vi "nanocal -- nuclear schottky fit V8.vi"() -> ()   [LabVIEW 2021] (continued)
   ,  \"mm3\" -> 0.162147674837   ,  \"T\" -> 0.178000000000   ,  \"B\" -> 8.000000000000   ,  \"θ\" -> 90.000000000000   ,  \"Reoff\" -> 0.000000000000   ,  \"Imoff\" -> 0.000000000000   ,  \"στ1\" -> 0.000050446338   ,  \"στS\" -> 0.000029155358   ,  \"στN\" -> 0.000054402622   ,  \"τ11 \" -> 0.000000000000   ,  \"τ12\" -> 0.000000000000   ,  \"τ22\" -> 0.000000000000   ,  \"τN1\" -> 0.000000000000   ,  \"τN2\" -> 0.000000000000   ,  \"σηlogτ1 \" -> 0.161173739457   ,  \"σηlogτS\" -> 0.007924149958   ,  \"σηlogτN\" -> 0.155365649649   ,  \"σlogτ1\" -> 0.001613673870   ,  \"σlogτS\" -> 0.000552329615   ,  \"σlogτN\" -> 0.000864292135   ,  \"σητ1\" -> 0.005038580001   ,  \"σητS \" -> 0.000418285426   ,  \"σητN\" -> 0.009779446506    |>   , \n\"IDS0348_210906_RAW_cal__sam_\" ->   <|    \"ζ\" -> 0.135783247929   ,  \"τ1\" -> 0.037121050091   ,  \"τS\" -> 0.079201640502   ,  \"τN\" -> 0.079201640502   ,  \"τC\" -> 0.001474311209   ,  \"κ0\" -> 0.000000000894   ,  \"mm1\" -> 0.000173730712   ,  \"mm2\" -> 0.016810842330   ,  \"mm3\" -> 0.201522581240   ,  \"T\" -> 0.178000000000   ,  \"B\" -> 8.000000000000   ,  \"θ\" -> 90.000000000000   ,  \"Reoff\" -> -29680722.891566276600   ,  \"Imoff\" -> 0.000000000000   ,  \"στ1\" -> 0.000000000000   ,  \"στS\" -> 0.000000000000   ,  \"στN\" -> 0.000000000000   ,  \"τ11 \" -> 0.000000000000   ,  \"τ12\" -> 0.000000000000   ,  \"τ22\" -> 0.000000000000   ,  \"τN1\" -> 0.000000000000   ,  \"τN2\" -> 0.000000000000   ,  \"σηlogτ1 \" -> 0.000000000000   ,  \"σηlogτS\" -> 0.000000000000   ,  \"σηlogτN\" -> 0.000000000000   ,  \"σlogτ1\" -> 0.000000000000   ,  \"σlogτS\" -> 0.000000000000   ,  \"σlogτN\" -> 0.000000000000   ,  \"σητ1\" -> 0.000000000000   ,  \"σητS \" -> 0.000000000000   ,  \"σητN\" -> 0.000000000000    |>   , \n\"IDS0349_210906_RAW_cal__ref_\" ->   <|    \"ζ\" -> 0.197057469427   ,  \"τ1\" -> 0.029613620558   ,  \"τS\" -> 0.050911815815   ,  \"τN\" -> 0.036816442025   ,  \"τC\" -> 0.000965034060   ,  \"κ0\" -> 0.000000001032   ,  \"mm1\" -> 0.000156774968   ,  \"mm2\" -> 0.015211417778   ,  \"mm3\" -> 0.120226228200   ,  \"T\" -> 0.200000000000   ,  \"B\" -> 8.000000000000   ,  \"θ\" -> 90.000000000000   ,  \"Reoff\" -> 0.000000000000   ,  \"Imoff\" -> 0.000000000000   ,  \"στ1\" -> 0.000057169127   ,  \"στS\" -> 0.000023609008   ,  \"στN\" -> 0.000037318979   ,  \"τ11 \" -> 0.000000000000   ,  \"τ12\" -> 0.000000000000   ,  \"τ22\" -> 0.000000000000   ,  \"τN1\" -> 0.000000000000   ,  \"τN2\" -> 0.000000000000   ,  \"σηlogτ1 \" -> 0.161376688793   ,  \"σηlogτS\" -> 0.005816962816   ,  \"σηlogτN\" -> 0.148995950079   ,  \"σlogτ1\" -> 0.001930501090   ,  \"σlogτS\" -> 0.000463723546   ,  \"σlogτN\" -> 0.001013649805   ,  \"σητ1\" -> 0.004778948029   ,  \"σητS \" -> 0.000296152139   ,  \"σητN\" -> 0.005485500758    |>   , \n\"IDS0349_210906_RAW_cal__sam_\" ->   <|    \"ζ\" -> 0.113690190882   ,  \"τ1\" -> 0.032691214581   ,  \"τS\" -> 0.068786957350   ,  \"τN\" -> 0.048058332081   ,  \"τC\" -> 0.001613875480   ,  \"κ0\" -> 0.000000001156   ,  \"mm1\" -> 0.000161675745   ,  \"mm2\" -> 0.017372504664   ,  \"mm3\" -> 0.146900362342   ,  \"T\" -> 0.200000000000   ,  \"B\" -> 8.000000000000   ,  \"θ\" -> 90.000000000000   ,  \"Reoff\" -> -14590361.445783138300   ,  \"Imoff\" -> 0.000000000000   ,  \"στ1\" -> 0.000000000000   ,  \"στS\" -> 0.000000000000   ,  \"στN\" -> 0.000000000000   ,  \"τ11 \" -> 0.000000000000   ,  \"τ12\" -> 0.000000000000   ,  \"τ22\" -> 0.000000000000   ,  \"τN1\" -> 0.000000000000   ,  \"τN2\" -> 0.000000000000   ,  \"σηlogτ1 \" -> 0.000000000000   ,  \"σηlogτS\" -> 0.000000000000   ,  \"σηlogτN\" -> 0.000000000000   ,  \"σlogτ1\" -> 0.000000000000   ,  \"σlogτS\" -> 0.000000000000   ,  \"σlogτN\" -> 0.000000000000   ,  \"σητ1\" -> 0.000000000000   ,  \"σητS \" -> 0.000000000000   ,  \"σητN\" -> 0.000000000000    |>   , \n\"IDS0350_210906_RAW_cal__ref_\" ->   <|    \"ζ\" -> 0.116383968065   ,  \"τ1\" -> 0.022837025685   ,  \"τS\" -> 0.041355624864   ,  \"τN\" -> 0.016243225582   ,  \"τC\" -> 0.001144746242   ,  \"κ0\" -> 0.000000001355   ,  \"mm1\" -> 0.000116736213   ,  \"mm2\" -> 0.014664448269   ,  \"mm3\" -> 0.073503020661   ,  \"T\" -> 0.260000000000   ,  \"B\" -> 8.000000000000   ,  \"θ\" -> 90.000000000000   ,  \"Reoff\" -> 0.000000000000   ,  \"Imoff\" -> 0.000000000000   ,  \"στ1\" -> 0.000027906584   ,  \"στS\" -> 0.000007380086   ,  \"στN\" -> 0.000010191855   ,  \"τ11 \" -> 0.000000000000   ,  \"τ12\" -> 0.000000000000   ,  \"τ22\" -> 0.000000000000   ,  \"τN1\" -> 0.000000000000   ,  \"τN2\" -> 0.000000000000   ,  \"σηlogτ1 \" -> 0.162256483080   ,  \"σηlogτS\" -> 0.003668520899   ,  \"σηlogτN\" -> 0.144232966841   ,  \"σlogτ1\" -> 0.001221988557   ,  \"σlogτS\" -> 0.000178454219   ,  \"σlogτN\" -> 0.000627452654   ,  \"σητ1\" -> 0.003705455472   ,  \"σητS \" -> 0.000151713974   ,  \"σητN\" -> 0.002342808617    |>   , \n\"IDS0350_210906_RAW_cal__sam_\" ->   <|    \"ζ\" -> 0.071614468485   ,  \"τ1\" -> 0.024327525692   ,  \"τS\" -> 0.055056024171   ,  \"τN\" -> 0.019709093999   ,  \"τC\" -> 0.001754398678   ,  \"κ0\" -> 0.000000001497   ,  \"mm1\" -> 0.000114067222   ,  \"mm2\" -> 0.016460052715   ,  \"mm3\" -> 0.089627186802   ,  \"T\" -> 0.260000000000   ,  \"B\" -> 8.000000000000   ,  \"θ\" -> 90.000000000000   ,  \"Reoff\" -> -10063253.012048184900   ,  \"Imoff\" -> 0.000000000000   ,  \"στ1\" -> 0.000000000000   ,  \"στS\" -> 0.000000000000   ,  \"στN\" -> 0.000000000000   ,  \"τ11 \" -> 0.000000000000   ,  \"τ12\" -> 0.000000000000   ,  \"τ22\" -> 0.000000000000   ,  \"τN1\" -> 0.000000000000   ,  \"τN2\" -> 0.000000000000   ,  \"σηlogτ1 \" -> 0.000000000000   ,  \"σηlogτS\" -> 0.000000000000   ,  \"σηlogτN\" -> 0.000000000000   ,  \"σlogτ1\" -> 0.000000000000   ,  \"σlogτS\" -> 0.000000000000   ,  \"σlogτN\" -> 0.000000000000   ,  \"σητ1\" -> 0.000000000000   ,  \"σητS \" -> 0.000000000000   ,  \"σητN\" -> 0.000000000000    |>   , \n\"IDS0351_210906_RAW_cal__ref_\" ->   <|    \"ζ\" -> 0.080064937947   ,  \"τ1\" -> 0.017296327437   ,  \"τS\" -> 0.036479707086   ,  \"τN\" -> 0.008116806938   ,  \"τC\" -> 0.001346314476   ,  \"κ0\" -> 0.000000001766   ,  \"mm1\" -> 0.000096730306   ,  \"mm2\" -> 0.013119572666   ,  \"mm3\" -> 0.053593470093   ,  \"T\" -> 0.310000000000   ,  \"B\" -> 8.000000000000   ,  \"θ\" -> 90.000000000000   ,  \"Reoff\" -> 0.000000000000   ,  \"Imoff\" -> 0.000000000000   ,  \"στ1\" -> 0.000031102743   ,  \"στS\" -> 0.000006077841   ,  \"στN\" -> 0.000007305969   ,  \"τ11 \" -> 0.000000000000   ,  \"τ12\" -> 0.000000000000   ,  \"τ22\" -> 0.000000000000   ,  \"τN1\" -> 0.000000000000   ,  \"τN2\" -> 0.000000000000   ,  \"σηlogτ1 \" -> 0.176104217691   ,  \"σηlogτS\" -> 0.002693810692   ,  \"σηlogτN\" -> 0.144358868609   ,  \"σlogτ1\" -> 0.001798228177   ,  \"σlogτS\" -> 0.000166608817   ,  \"σlogτN\" -> 0.000900103833   ,  \"σητ1\" -> 0.003045956212   ,  \"σητS \" -> 0.000098269425   ,  \"σητN\" -> 0.001171733066    |>   , \n\"IDS0351_210906_RAW_cal__sam_\" ->   <|    \"ζ\" -> 0.049866383839   ,  \"τ1\" -> 0.023285662985   ,  \"τS\" -> 0.049370833464   ,  \"τN\" -> 0.009866658615   ,  \"τC\" -> 0.002153040267   ,  \"κ0\" -> 0.000000001928   ,  \"mm1\" -> 0.000098362318   ,  \"mm2\" -> 0.018063601956   ,  \"mm3\" -> 0.069468190575   ,  \"T\" -> 0.310000000000   ,  \"B\" -> 8.000000000000   ,  \"θ\" -> 90.000000000000   ,  \"Reoff\" -> -5536144.578313261270   ,  \"Imoff\" -> 0.000000000000   ,  \"στ1\" -> 0.000000000000   ,  \"στS\" -> 0.000000000000   ,  \"στN\" -> 0.000000000000   ,  \"τ11 \" -> 0.000000000000   ,  \"τ12\" -> 0.000000000000   ,  \"τ22\" -> 0.000000000000   ,  \"τN1\" -> 0.000000000000   ,  \"τN2\" -> 0.000000000000   ,  \"σηlogτ1 \" -> 0.000000000000   ,  \"σηlogτS\" -> 0.000000000000   ,  \"σηlogτN\" -> 0.000000000000   ,  \"σlogτ1\" -> 0.000000000000   ,  \"σlogτS\" -> 0.000000000000   ,  \"σlogτN\" -> 0.000000000000   ,  \"σητ1\" -> 0.000000000000   ,  \"σητS \" -> 0.000000000000   ,  \"σητN\" -> 0.000000000000    |>   , \n\"IDS0352_210906_RAW_cal__ref_\" ->   <|    \"ζ\" -> 0.060178216595   ,  \"τ1\" -> 0.015538327560   ,  \"τS\" -> 0.033922393417   ,  \"τN\" -> 0.005018769313   ,  \"τC\" -> 0.001649636137   ,  \"κ0\" -> 0.000000002110   ,  \"mm1\" -> 0.000089741441   ,  \"mm2\" -> 0.012788298806   ,  \"mm3\" -> 0.045594495906   ,  \"T\" -> 0.360000000000   ,  \"B\" -> 8.000000000000   ,  \"θ\" -> 90.000000000000   ,  \"Reoff\" -> 0.000000000000   ,  \"Imoff\" -> 0.000000000000   ,  \"στ1\" -> 0.000024762200   ,  \"στS\" -> 0.000003463726   ,  \"στN\" -> 0.000003978144   ,  \"τ11 \" -> 0.000000000000   ,  \"τ12\" -> 0.000000000000   ,  \"τ22\" -> 0.000000000000   ,  \"τN1\" -> 0.000000000000   ,  \"τN2\" -> 0.000000000000   ,  \"σηlogτ1 \" -> 0.179978131634   ,  \"σηlogτS\" -> 0.001942969644   ,  \"σηlogτN\" -> 0.143630935441   ,  \"σlogτ1\" -> 0.001593620678   ,  \"σlogτS\" -> 0.000102107372   ,  \"σlogτN\" -> 0.000792653332   ,  \"σητ1\" -> 0.002796559163   ,  \"σητS \" -> 0.000065910181   ,  \"σητN\" -> 0.000720850531    |>   , \n\"IDS0352_210906_RAW_cal__sam_\" ->   <|    \"ζ\" -> 0.036116393265   ,  \"τ1\" -> 0.020310974732   ,  \"τS\" -> 0.044594628397   ,  \"τN\" -> 0.005932938101   ,  \"τC\" -> 0.002747123875   ,  \"κ0\" -> 0.000000002292   ,  \"mm1\" -> 0.000090548575   ,  \"mm2\" -> 0.017024776182   ,  \"mm3\" -> 0.058295213810   ,  \"T\" -> 0.360000000000   ,  \"B\" -> 8.000000000000   ,  \"θ\" -> 90.000000000000   ,  \"Reoff\" -> -2518072.289156645540   ,  \"Imoff\" -> 0.000000000000   ,  \"στ1\" -> 0.000000000000   ,  \"στS\" -> 0.000000000000   ,  \"στN\" -> 0.000000000000   ,  \"τ11 \" -> 0.000000000000   ,  \"τ12\" -> 0.000000000000   ,  \"τ22\" -> 0.000000000000   ,  \"τN1\" -> 0.000000000000   ,  \"τN2\" -> 0.000000000000   ,  \"σηlogτ1 \" -> 0.000000000000   ,  \"σηlogτS\" -> 0.000000000000   ,  \"σηlogτN\" -> 0.000000000000   ,  \"σlogτ1\" -> 0.000000000000   ,  \"σlogτS\" -> 0.000000000000   ,  \"σlogτN\" -> 0.000000000000   ,  \"σητ1\" -> 0.000000000000   ,  \"σητS \" -> 0.000000000000   ,  \"σητN\" -> 0.000000000000    |>   , \n\"IDS0353_210906_RAW_cal__ref_\" ->   <|    \"ζ\" -> 0.043805011586   ,  \"τ1\" -> 0.015641832651   ,  \"τS\" -> 0.031297289619   ,  \"τN\" -> 0.002720036846   ,  \"τC\" -> 0.001830581120   ,  \"κ0\" -> 0.000000002632   ,  \"mm1\" -> 0.000072899501   ,  \"mm2\" -> 0.013753455926   ,  \"mm3\" -> 0.039153514190   ,  \"T\" -> 0.438000000000   ,  \"B\" -> 8.000000000000   ,  \"θ\" -> 90.000000000000   ,  \"Reoff\" -> 0.000000000000   ,  \"Imoff\" -> 0.000000000000   ,  \"στ1\" -> 0.000029789904   ,  \"στS\" -> 0.000002213568   ,  \"στN\" -> 0.000002569992   ,  \"τ11 \" -> 0.000000000000   ,  \"τ12\" -> 0.000000000000   ,  \"τ22\" -> 0.000000000000   ,  \"τN1\" -> 0.000000000000   ,  \"τN2\" -> 0.000000000000   ,  \"σηlogτ1 \" -> 0.171230545078   ,  \"σηlogτS\" -> 0.001043214583   ,  \"σηlogτN\" -> 0.141039696626   ,  \"σlogτ1\" -> 0.001904502144   ,  \"σlogτS\" -> 0.000070727156   ,  \"σlogτN\" -> 0.000944837375   ,  \"σητ1\" -> 0.002678359531   ,  \"σητS \" -> 0.000032649789   ,  \"σητN\" -> 0.000383633172    |>   , \n\"IDS0353_210906_RAW_cal__sam_\" ->   <|    \"ζ\" -> 0.028235631162   ,  \"τ1\" -> 0.018033623612   ,  \"τS\" -> 0.040112967891   ,  \"τN\" -> 0.003332308168   ,  \"τC\" -> 0.002994357278   ,  \"κ0\" -> 0.000000002859   ,  \"mm1\" -> 0.000076791949   ,  \"mm2\" -> 0.016073609718   ,  \"mm3\" -> 0.049549560072   ,  \"T\" -> 0.438000000000   ,  \"B\" -> 8.000000000000   ,  \"θ\" -> 90.000000000000   ,  \"Reoff\" -> -2200000.000000000000   ,  \"Imoff\" -> 0.000000000000   ,  \"στ1\" -> 0.000000000000   ,  \"στS\" -> 0.000000000000   ,  \"στN\" -> 0.000000000000   ,  \"τ11 \" -> 0.000000000000   ,  \"τ12\" -> 0.000000000000   ,  \"τ22\" -> 0.000000000000   ,  \"τN1\" -> 0.000000000000   ,  \"τN2\" -> 0.000000000000   ,  \"σηlogτ1 \" -> 0.000000000000   ,  \"σηlogτS\" -> 0.000000000000   ,  \"σηlogτN\" -> 0.000000000000   ,  \"σlogτ1\" -> 0.000000000000   ,  \"σlogτS\" -> 0.000000000000   ,  \"σlogτN\" -> 0.000000000000   ,  \"σητ1\" -> 0.000000000000   ,  \"σητS \" -> 0.000000000000   ,  \"σητN\" -> 0.000000000000    |>   , \n\"IDS0354_210906_RAW_cal__ref_\" ->   <|    \"ζ\" -> 0.034407438278   ,  \"τ1\" -> 0.012759993552   ,  \"τS\" -> 0.028549472180   ,  \"τN\" -> 0.001373973335   ,  \"τC\" -> 0.002126234468   ,  \"κ0\" -> 0.000000003285   ,  \"mm1\" -> 0.000066111743   ,  \"mm2\" -> 0.011901304001   ,  \"mm3\" -> 0.033871846896   ,  \"T\" -> 0.530000000000   ,  \"B\" -> 8.000000000000   ,  \"θ\" -> 90.000000000000   ,  \"Reoff\" -> 0.000000000000   ,  \"Imoff\" -> 0.000000000000   ,  \"στ1\" -> 0.000105401331   ,  \"στS\" -> 0.000005152140   ,  \"στN\" -> 0.000005607099   ,  \"τ11 \" -> 0.000000000000   ,  \"τ12\" -> 0.000000000000   ,  \"τ22\" -> 0.000000000000   ,  \"τN1\" -> 0.000000000000   ,  \"τN2\" -> 0.000000000000   ,  \"σηlogτ1 \" -> 0.184333164792   ,  \"σηlogτS\" -> 0.000694064017   ,  \"σηlogτN\" -> 0.142381877257   ,  \"σlogτ1\" -> 0.008260296568   ,  \"σlogτS\" -> 0.000180463565   ,  \"σlogτN\" -> 0.004080937594   ,  \"σητ1\" -> 0.002352089994   ,  \"σητS \" -> 0.000019815161   ,  \"σητN\" -> 0.000195628903    |>   , \n\"IDS0354_210906_RAW_cal__sam_\" ->   <|    \"ζ\" -> 0.022962333090   ,  \"τ1\" -> 0.020865157142   ,  \"τS\" -> 0.035948400917   ,  \"τN\" -> 0.001990138096   ,  \"τC\" -> 0.003574397791   ,  \"κ0\" -> 0.000000003542   ,  \"mm1\" -> 0.000073258085   ,  \"mm2\" -> 0.019040364220   ,  \"mm3\" -> 0.044135629011   ,  \"T\" -> 0.530000000000   ,  \"B\" -> 8.000000000000   ,  \"θ\" -> 90.000000000000   ,  \"Reoff\" -> -1700000.000000000000   ,  \"Imoff\" -> 0.000000000000   ,  \"στ1\" -> 0.000000000000   ,  \"στS\" -> 0.000000000000   ,  \"στN\" -> 0.000000000000   ,  \"τ11 \" -> 0.000000000000   ,  \"τ12\" -> 0.000000000000   ,  \"τ22\" -> 0.000000000000   ,  \"τN1\" -> 0.000000000000   ,  \"τN2\" -> 0.000000000000   ,  \"σηlogτ1 \" -> 0.000000000000   ,  \"σηlogτS\" -> 0.000000000000   ,  \"σηlogτN\" -> 0.000000000000   ,  \"σlogτ1\" -> 0.000000000000   ,  \"σlogτS\" -> 0.000000000000   ,  \"σlogτN\" -> 0.000000000000   ,  \"σητ1\" -> 0.000000000000   ,  \"σητS \" -> 0.000000000000   ,  \"σητN\" -> 0.000000000000    |>   , \n\"IDS0355_210906_RAW_cal__ref_\" ->   <|    \"ζ\" -> 0.020775547522   ,  \"τ1\" -> 0.014245155504   ,  \"τS\" -> 0.021871141548   ,  \"τN\" -> 0.000446024292   ,  \"τC\" -> 0.003241636501   ,  \"κ0\" -> 0.000000005421   ,  \"mm1\" -> 0.000057740843   ,  \"mm2\" -> 0.013715964924   ,  \"mm3\" -> 0.026493903417   ,  \"T\" -> 0.830000000000   ,  \"B\" -> 8.000000000000   ,  \"θ\" -> 90.000000000000   ,  \"Reoff\" -> 0.000000000000   ,  \"Imoff\" -> 0.000000000000   ,  \"στ1\" -> 0.000172291727   ,  \"στS\" -> 0.000002161761   ,  \"στN\" -> 0.000002696691   ,  \"τ11 \" -> 0.000000000000   ,  \"τ12\" -> 0.000000000000   ,  \"τ22\" -> 0.000000000000   ,  \"τN1\" -> 0.000000000000   ,  \"τN2\" -> 0.000000000000   ,  \"σηlogτ1 \" -> 0.152304599872   ,  \"σηlogτS\" -> 0.000189712528   ,  \"σηlogτN\" -> 0.136839329472   ,  \"σlogτ1\" -> 0.012094759326   ,  \"σlogτS\" -> 0.000098840802   ,  \"σlogτN\" -> 0.006046063343   ,  \"σητ1\" -> 0.002169602709   ,  \"σητS \" -> 0.000004149230   ,  \"σητN\" -> 0.000061033665    |>   , \n\"IDS0355_210906_RAW_cal__sam_\" ->   <|    \"ζ\" -> 0.015987398390   ,  \"τ1\" -> 0.023974349678   ,  \"τS\" -> 0.025824294014   ,  \"τN\" -> 0.000573136357   ,  \"τC\" -> 0.005688548480   ,  \"κ0\" -> 0.000000005865   ,  \"mm1\" -> 0.000073733721   ,  \"mm2\" -> 0.022561297233   ,  \"mm3\" -> 0.033847323811   ,  \"T\" -> 0.830000000000   ,  \"B\" -> 8.000000000000   ,  \"θ\" -> 90.000000000000   ,  \"Reoff\" -> -599999.999999999999   ,  \"Imoff\" -> 0.000000000000   ,  \"στ1\" -> 0.000000000000   ,  \"στS\" -> 0.000000000000   ,  \"στN\" -> 0.000000000000   ,  \"τ11 \" -> 0.000000000000   ,  \"τ12\" -> 0.000000000000   ,  \"τ22\" -> 0.000000000000   ,  \"τN1\" -> 0.000000000000   ,  \"τN2\" -> 0.000000000000   ,  \"σηlogτ1 \" -> 0.000000000000   ,  \"σηlogτS\" -> 0.000000000000   ,  \"σηlogτN\" -> 0.000000000000   ,  \"σlogτ1\" -> 0.000000000000   ,  \"σlogτS\" -> 0.000000000000   ,  \"σlogτN\" -> 0.000000000000   ,  \"σητ1\" -> 0.000000000000   ,  \"σητS \" -> 0.000000000000   ,  \"σητN\" -> 0.000000000000    |>   , \n\"IDS0359_210907_RAW_cal__ref_\" ->   <|    \"ζ\" -> 0.424845059741   ,  \"τ1\" -> 0.089321051678   ,  \"τS\" -> 0.116595960023   ,  \"τN\" -> 0.612122896867   ,  \"τC\" -> 0.001120095408   ,  \"κ0\" -> 0.000000000383   ,  \"mm1\" -> 0.000332370585   ,  \"mm2\" -> 0.013372321421   ,  \"mm3\" -> 1.115047918259   ,  \"T\" -> 0.120000000000   ,  \"B\" -> 12.000000000000   ,  \"θ\" -> 60.000000000000   ,  \"Reoff\" -> 0.000000000000   ,  \"Imoff\" -> 0.000000000000   ,  \"στ1\" -> 0.000839647107   ,  \"στS\" -> 0.000700328201   ,  \"στN\" -> 0.003352050812   ,  \"τ11 \" -> 0.000000000000   ,  \"τ12\" -> 0.000000000000   ,  \"τ22\" -> 0.000000000000   ,  \"τN1\" -> 0.000000000000   ,  \"τN2\" -> 0.000000000000   ,  \"σηlogτ1 \" -> 0.058996717292   ,  \"σηlogτS\" -> 0.003693056048   ,  \"σηlogτN\" -> 0.066658525220   ,  \"σlogτ1\" -> 0.009400327147   ,  \"σlogτS\" -> 0.006006453401   ,  \"σlogτN\" -> 0.005476107542   ,  \"σητ1\" -> 0.005269648834   ,  \"σητS \" -> 0.000430595415   ,  \"σητN\" -> 0.040803209559    |>   , \n\"IDS0359_210907_RAW_cal__sam_\" ->   <|    \"ζ\" -> 0.241762987309   ,  \"τ1\" -> 0.090301757431   ,  \"τS\" -> 0.104468976957   ,  \"τN\" -> 0.810352557873   ,  \"τC\" -> 0.001702208121   ,  \"κ0\" -> 0.000000000500   ,  \"mm1\" -> 0.000327834342   ,  \"mm2\" -> 0.009723084216   ,  \"mm3\" -> 1.217944568939   ,  \"T\" -> 0.120000000000   ,  \"B\" -> 12.000000000000   ,  \"θ\" -> 60.000000000000   ,  \"Reoff\" -> -52289156.626506023100   ,  \"Imoff\" -> 0.000000000000   ,  \"στ1\" -> 0.000000000000   ,  \"στS\" -> 0.000000000000   ,  \"στN\" -> 0.000000000000   ,  \"τ11 \" -> 0.000000000000   ,  \"τ12\" -> 0.000000000000   ,  \"τ22\" -> 0.000000000000   ,  \"τN1\" -> 0.000000000000   ,  \"τN2\" -> 0.000000000000   ,  \"σηlogτ1 \" -> 0.000000000000   ,  \"σηlogτS\" -> 0.000000000000   ,  \"σηlogτN\" -> 0.000000000000   ,  \"σlogτ1\" -> 0.000000000000   ,  \"σlogτS\" -> 0.000000000000   ,  \"σlogτN\" -> 0.000000000000   ,  \"σητ1\" -> 0.000000000000   ,  \"σητS \" -> 0.000000000000   ,  \"σητN\" -> 0.000000000000    |>   , \n\"IDS0360_210907_RAW_cal__ref_\" ->   <|    \"ζ\" -> 0.342434399581   ,  \"τ1\" -> 0.078890152129   ,  \"τS\" -> 0.062757285209   ,  \"τN\" -> 0.289377193045   ,  \"τC\" -> 0.000956599249   ,  \"κ0\" -> 0.000000000628   ,  \"mm1\" -> 0.000241931953   ,  \"mm2\" -> 0.012416031233   ,  \"mm3\" -> 0.539906225078   ,  \"T\" -> 0.150000000000   ,  \"B\" -> 12.000000000000   ,  \"θ\" -> 60.000000000000   ,  \"Reoff\" -> 0.000000000000   ,  \"Imoff\" -> 0.000000000000   ,  \"στ1\" -> 0.000259479640   ,  \"στS\" -> 0.000106061605   ,  \"στN\" -> 0.000644908503   ,  \"τ11 \" -> 0.000000000000   ,  \"τ12\" -> 0.000000000000   ,  \"τ22\" -> 0.000000000000   ,  \"τN1\" -> 0.000000000000   ,  \"τN2\" -> 0.000000000000   ,  \"σηlogτ1 \" -> 0.046682907310   ,  \"σηlogτS\" -> 0.002342389923   ,  \"σηlogτN\" -> 0.056973626918   ,  \"σlogτ1\" -> 0.003289125866   ,  \"σlogτS\" -> 0.001690028567   ,  \"σlogτN\" -> 0.002228608605   ,  \"σητ1\" -> 0.003682821660   ,  \"σητS \" -> 0.000147002032   ,  \"σητN\" -> 0.016486868235    |>   , \n\"IDS0360_210907_RAW_cal__sam_\" ->   <|    \"ζ\" -> 0.201278537585   ,  \"τ1\" -> 0.081544073952   ,  \"τS\" -> 0.088995303529   ,  \"τN\" -> 0.405130496924   ,  \"τC\" -> 0.001460686320   ,  \"κ0\" -> 0.000000000739   ,  \"mm1\" -> 0.000241947199   ,  \"mm2\" -> 0.013299947862   ,  \"mm3\" -> 0.663045584163   ,  \"T\" -> 0.150000000000   ,  \"B\" -> 12.000000000000   ,  \"θ\" -> 60.000000000000   ,  \"Reoff\" -> -39048192.771084338400   ,  \"Imoff\" -> 0.000000000000   ,  \"στ1\" -> 0.000000000000   ,  \"στS\" -> 0.000000000000   ,  \"στN\" -> 0.000000000000   ,  \"τ11 \" -> 0.000000000000   ,  \"τ12\" -> 0.000000000000   ,  \"τ22\" -> 0.000000000000   ,  \"τN1\" -> 0.000000000000   ,  \"τN2\" -> 0.000000000000   ,  \"σηlogτ1 \" -> 0.000000000000   ,  \"σηlogτS\" -> 0.000000000000   ,  \"σηlogτN\" -> 0.000000000000   ,  \"σlogτ1\" -> 0.000000000000   ,  \"σlogτS\" -> 0.000000000000   ,  \"σlogτN\" -> 0.000000000000   ,  \"σητ1\" -> 0.000000000000   ,  \"σητS \" -> 0.000000000000   ,  \"σητN\" -> 0.000000000000    |>   , \n\"IDS0361_210908_RAW_cal__ref_\" ->   <|    \"ζ\" -> 0.274843315726   ,  \"τ1\" -> 0.065669556126   ,  \"τS\" -> 0.043737045326   ,  \"τN\" -> 0.171424826572   ,  \"τC\" -> 0.000899266573   ,  \"κ0\" -> 0.000000000755   ,  \"mm1\" -> 0.000191414578   ,  \"mm2\" -> 0.011258128300   ,  \"mm3\" -> 0.329416954010   ,  \"T\" -> 0.168000000000   ,  \"B\" -> 12.000000000000   ,  \"θ\" -> 60.000000000000   ,  \"Reoff\" -> 0.000000000000   ,  \"Imoff\" -> 0.000000000000   ,  \"στ1\" -> 0.000077610156   ,  \"στS\" -> 0.000022738638   ,  \"στN\" -> 0.000144137782   ,  \"τ11 \" -> 0.000000000000   ,  \"τ12\" -> 0.000000000000   ,  \"τ22\" -> 0.000000000000   ,  \"τN1\" -> 0.000000000000   ,  \"τN2\" -> 0.000000000000   ,  \"σηlogτ1 \" -> 0.041134517971   ,  \"σηlogτS\" -> 0.001768570492   ,  \"σηlogτN\" -> 0.052373530031   ,  \"σlogτ1\" -> 0.001181828544   ,  \"σlogτS\" -> 0.000519894231   ,  \"σlogτN\" -> 0.000840822097   ,  \"σητ1\" -> 0.002701285537   ,  \"σητS \" -> 0.000077352048   ,  \"σητN\" -> 0.008978123302    |>   , \n\"IDS0361_210908_RAW_cal__sam_\" ->   <|    \"ζ\" -> 0.166104690940   ,  \"τ1\" -> 0.071049175548   ,  \"τS\" -> 0.068661809155   ,  \"τN\" -> 0.222482953546   ,  \"τC\" -> 0.001364223445   ,  \"κ0\" -> 0.000000000861   ,  \"mm1\" -> 0.000191495940   ,  \"mm2\" -> 0.014533832786   ,  \"mm3\" -> 0.397193343795   ,  \"T\" -> 0.168000000000   ,  \"B\" -> 12.000000000000   ,  \"θ\" -> 60.000000000000   ,  \"Reoff\" -> -34789156.626506023100   ,  \"Imoff\" -> 0.000000000000   ,  \"στ1\" -> 0.000000000000   ,  \"στS\" -> 0.000000000000   ,  \"στN\" -> 0.000000000000   ,  \"τ11 \" -> 0.000000000000   ,  \"τ12\" -> 0.000000000000   ,  \"τ22\" -> 0.000000000000   ,  \"τN1\" -> 0.000000000000   ,  \"τN2\" -> 0.000000000000   ,  \"σηlogτ1 \" -> 0.000000000000   ,  \"σηlogτS\" -> 0.000000000000   ,  \"σηlogτN\" -> 0.000000000000   ,  \"σlogτ1\" -> 0.000000000000   ,  \"σlogτS\" -> 0.000000000000   ,  \"σlogτN\" -> 0.000000000000   ,  \"σητ1\" -> 0.000000000000   ,  \"σητS \" -> 0.000000000000   ,  \"σητN\" -> 0.000000000000    |>   , \n\"IDS0362_210908_RAW_cal__ref_\" ->   <|    \"ζ\" -> 0.210826162252   ,  \"τ1\" -> 0.054763021259   ,  \"τS\" -> 0.037603010957   ,  \"τN\" -> 0.089871422671   ,  \"τC\" -> 0.000959483183   ,  \"κ0\" -> 0.000000001045   ,  \"mm1\" -> 0.000164174443   ,  \"mm2\" -> 0.012877562256   ,  \"mm3\" -> 0.197030146997   ,  \"T\" -> 0.197000000000   ,  \"B\" -> 12.000000000000   ,  \"θ\" -> 60.000000000000   ,  \"Reoff\" -> 0.000000000000   ,  \"Imoff\" -> 0.000000000000   ,  \"στ1\" -> 0.000049220168   ,  \"στS\" -> 0.000011686979   ,  \"στN\" -> 0.000056446769   ,  \"τ11 \" -> 0.000000000000   ,  \"τ12\" -> 0.000000000000   ,  \"τ22\" -> 0.000000000000   ,  \"τN1\" -> 0.000000000000   ,  \"τN2\" -> 0.000000000000   ,  \"σηlogτ1 \" -> 0.038148915938   ,  \"σηlogτS\" -> 0.001374810052   ,  \"σηlogτN\" -> 0.048522876787   ,  \"σlogτ1\" -> 0.000898784750   ,  \"σlogτS\" -> 0.000310799031   ,  \"σlogτN\" -> 0.000628083622   ,  \"σητ1\" -> 0.002089149895   ,  \"σητS \" -> 0.000051696997   ,  \"σητN\" -> 0.004360819969    |>   , \n\"IDS0362_210908_RAW_cal__sam_\" ->   <|    \"ζ\" -> 0.123741217510   ,  \"τ1\" -> 0.059103977068   ,  \"τS\" -> 0.051096152058   ,  \"τN\" -> 0.122661863704   ,  \"τC\" -> 0.001502836172   ,  \"κ0\" -> 0.000000001149   ,  \"mm1\" -> 0.000161683871   ,  \"mm2\" -> 0.014394250129   ,  \"mm3\" -> 0.241309923424   ,  \"T\" -> 0.197000000000   ,  \"B\" -> 12.000000000000   ,  \"θ\" -> 60.000000000000   ,  \"Reoff\" -> -17448795.180722892300   ,  \"Imoff\" -> 0.000000000000   ,  \"στ1\" -> 0.000000000000   ,  \"στS\" -> 0.000000000000   ,  \"στN\" -> 0.000000000000   ,  \"τ11 \" -> 0.000000000000   ,  \"τ12\" -> 0.000000000000   ,  \"τ22\" -> 0.000000000000   ,  \"τN1\" -> 0.000000000000   ,  \"τN2\" -> 0.000000000000   ,  \"σηlogτ1 \" -> 0.000000000000   ,  \"σηlogτS\" -> 0.000000000000   ,  \"σηlogτN\" -> 0.000000000000   ,  \"σlogτ1\" -> 0.000000000000   ,  \"σlogτS\" -> 0.000000000000   ,  \"σlogτN\" -> 0.000000000000   ,  \"σητ1\" -> 0.000000000000   ,  \"σητS \" -> 0.000000000000   ,  \"σητN\" -> 0.000000000000    |>   , \n\"IDS0363_210908_RAW_cal__ref_\" ->   <|    \"ζ\" -> 0.120195011159   ,  \"τ1\" -> 0.037982415348   ,  \"τS\" -> 0.029921195592   ,  \"τN\" -> 0.032714371407   ,  \"τC\" -> 0.001103711032   ,  \"κ0\" -> 0.000000001361   ,  \"mm1\" -> 0.000115022123   ,  \"mm2\" -> 0.013740329759   ,  \"mm3\" -> 0.095394824172   ,  \"T\" -> 0.250000000000   ,  \"B\" -> 12.000000000000   ,  \"θ\" -> 60.000000000000   ,  \"Reoff\" -> 0.000000000000   ,  \"Imoff\" -> 0.000000000000   ,  \"στ1\" -> 0.000012313434   ,  \"στS\" -> 0.000002128775   ,  \"στN\" -> 0.000006964176   ,  \"τ11 \" -> 0.000000000000   ,  \"τ12\" -> 0.000000000000   ,  \"τ22\" -> 0.000000000000   ,  \"τN1\" -> 0.000000000000   ,  \"τN2\" -> 0.000000000000   ,  \"σηlogτ1 \" -> 0.037050900153   ,  \"σηlogτS\" -> 0.000901906922   ,  \"σηlogτN\" -> 0.045689519095   ,  \"σlogτ1\" -> 0.000324187744   ,  \"σlogτS\" -> 0.000071146055   ,  \"σlogτN\" -> 0.000212878182   ,  \"σητ1\" -> 0.001407282679   ,  \"σητS \" -> 0.000026986133   ,  \"σητN\" -> 0.001494703897    |>   , \n\"IDS0363_210908_RAW_cal__sam_\" ->   <|    \"ζ\" -> 0.074359211271   ,  \"τ1\" -> 0.044477620306   ,  \"τS\" -> 0.040449563551   ,  \"τN\" -> 0.044745540249   ,  \"τC\" -> 0.001712765821   ,  \"κ0\" -> 0.000000001493   ,  \"mm1\" -> 0.000114327803   ,  \"mm2\" -> 0.016556677808   ,  \"mm3\" -> 0.121049525039   ,  \"T\" -> 0.250000000000   ,  \"B\" -> 12.000000000000   ,  \"θ\" -> 60.000000000000   ,  \"Reoff\" -> -10147590.361445784600   ,  \"Imoff\" -> 0.000000000000   ,  \"στ1\" -> 0.000000000000   ,  \"στS\" -> 0.000000000000   ,  \"στN\" -> 0.000000000000   ,  \"τ11 \" -> 0.000000000000   ,  \"τ12\" -> 0.000000000000   ,  \"τ22\" -> 0.000000000000   ,  \"τN1\" -> 0.000000000000   ,  \"τN2\" -> 0.000000000000   ,  \"σηlogτ1 \" -> 0.000000000000   ,  \"σηlogτS\" -> 0.000000000000   ,  \"σηlogτN\" -> 0.000000000000   ,  \"σlogτ1\" -> 0.000000000000   ,  \"σlogτS\" -> 0.000000000000   ,  \"σlogτN\" -> 0.000000000000   ,  \"σητ1\" -> 0.000000000000   ,  \"σητS \" -> 0.000000000000   ,  \"σητN\" -> 0.000000000000    |>   , \n\"IDS0364_210908_RAW_cal__ref_\" ->   <|    \"ζ\" -> 0.081935948170   ,  \"τ1\" -> 0.032287614632   ,  \"τS\" -> 0.026949270434   ,  \"τN\" -> 0.016861876648   ,  \"τC\" -> 0.001338410345   ,  \"κ0\" -> 0.000000001744   ,  \"mm1\" -> 0.000097212898   ,  \"mm2\" -> 0.014855671361   ,  \"mm3\" -> 0.066073995677   ,  \"T\" -> 0.307000000000   ,  \"B\" -> 12.000000000000   ,  \"θ\" -> 60.000000000000   ,  \"Reoff\" -> 0.000000000000   ,  \"Imoff\" -> 0.000000000000   ,  \"στ1\" -> 0.000017118957   ,  \"στS\" -> 0.000002077535   ,  \"στN\" -> 0.000005632909   ,  \"τ11 \" -> 0.000000000000   ,  \"τ12\" -> 0.000000000000   ,  \"τ22\" -> 0.000000000000   ,  \"τN1\" -> 0.000000000000   ,  \"τN2\" -> 0.000000000000   ,  \"σηlogτ1 \" -> 0.036879495168   ,  \"σηlogτS\" -> 0.000607281388   ,  \"σηlogτN\" -> 0.044616936261   ,  \"σlogτ1\" -> 0.000530201983   ,  \"σlogτS\" -> 0.000077090575   ,  \"σlogτN\" -> 0.000334061782   ,  \"σητ1\" -> 0.001190750928   ,  \"σητS \" -> 0.000016365790   ,  \"σητN\" -> 0.000752325276    |>   , \n\"IDS0364_210908_RAW_cal__sam_\" ->   <|    \"ζ\" -> 0.051560123380   ,  \"τ1\" -> 0.037167172913   ,  \"τS\" -> 0.035875072163   ,  \"τN\" -> 0.021782945969   ,  \"τC\" -> 0.002191662682   ,  \"κ0\" -> 0.000000001902   ,  \"mm1\" -> 0.000101812126   ,  \"mm2\" -> 0.018093196790   ,  \"mm3\" -> 0.081794699340   ,  \"T\" -> 0.307000000000   ,  \"B\" -> 12.000000000000   ,  \"θ\" -> 60.000000000000   ,  \"Reoff\" -> -5584337.349397592250   ,  \"Imoff\" -> 0.000000000000   ,  \"στ1\" -> 0.000000000000   ,  \"στS\" -> 0.000000000000   ,  \"στN\" -> 0.000000000000   ,  \"τ11 \" -> 0.000000000000   ,  \"τ12\" -> 0.000000000000   ,  \"τ22\" -> 0.000000000000   ,  \"τN1\" -> 0.000000000000   ,  \"τN2\" -> 0.000000000000   ,  \"σηlogτ1 \" -> 0.000000000000   ,  \"σηlogτS\" -> 0.000000000000   ,  \"σηlogτN\" -> 0.000000000000   ,  \"σlogτ1\" -> 0.000000000000   ,  \"σlogτS\" -> 0.000000000000   ,  \"σlogτN\" -> 0.000000000000   ,  \"σητ1\" -> 0.000000000000   ,  \"σητS \" -> 0.000000000000   ,  \"σητN\" -> 0.000000000000    |>   , \n\"IDS0365_210908_RAW_cal__ref_\" ->   <|    \"ζ\" -> 0.060609447021   ,  \"τ1\" -> 0.026924433713   ,  \"τS\" -> 0.025092686079   ,  \"τN\" -> 0.009588284117   ,  \"τC\" -> 0.001648006453   ,  \"κ0\" -> 0.000000002119   ,  \"mm1\" -> 0.000088958851   ,  \"mm2\" -> 0.015130564959   ,  \"mm3\" -> 0.050135880977   ,  \"T\" -> 0.360000000000   ,  \"B\" -> 12.000000000000   ,  \"θ\" -> 60.000000000000   ,  \"Reoff\" -> 0.000000000000   ,  \"Imoff\" -> 0.000000000000   ,  \"στ1\" -> 0.000013873165   ,  \"στS\" -> 0.000001316641   ,  \"στN\" -> 0.000002948025   ,  \"τ11 \" -> 0.000000000000   ,  \"τ12\" -> 0.000000000000   ,  \"τ22\" -> 0.000000000000   ,  \"τN1\" -> 0.000000000000   ,  \"τN2\" -> 0.000000000000   ,  \"σηlogτ1 \" -> 0.038447991520   ,  \"σηlogτS\" -> 0.000466260948   ,  \"σηlogτN\" -> 0.044499975786   ,  \"σlogτ1\" -> 0.000515263014   ,  \"σlogτS\" -> 0.000052471110   ,  \"σlogτN\" -> 0.000307461145   ,  \"σητ1\" -> 0.001035190399   ,  \"σητS \" -> 0.000011699740   ,  \"σητN\" -> 0.000426678411    |>   , \n\"IDS0365_210908_RAW_cal__sam_\" ->   <|    \"ζ\" -> 0.037527154631   ,  \"τ1\" -> 0.031791574880   ,  \"τS\" -> 0.032568278603   ,  \"τN\" -> 0.012463984296   ,  \"τC\" -> 0.002682405917   ,  \"κ0\" -> 0.000000002306   ,  \"mm1\" -> 0.000090102201   ,  \"mm2\" -> 0.018466994147   ,  \"mm3\" -> 0.062639080041   ,  \"T\" -> 0.360000000000   ,  \"B\" -> 12.000000000000   ,  \"θ\" -> 60.000000000000   ,  \"Reoff\" -> -2846385.542168676850   ,  \"Imoff\" -> 0.000000000000   ,  \"στ1\" -> 0.000000000000   ,  \"στS\" -> 0.000000000000   ,  \"στN\" -> 0.000000000000   ,  \"τ11 \" -> 0.000000000000   ,  \"τ12\" -> 0.000000000000   ,  \"τ22\" -> 0.000000000000   ,  \"τN1\" -> 0.000000000000   ,  \"τN2\" -> 0.000000000000   ,  \"σηlogτ1 \" -> 0.000000000000   ,  \"σηlogτS\" -> 0.000000000000   ,  \"σηlogτN\" -> 0.000000000000   ,  \"σlogτ1\" -> 0.000000000000   ,  \"σlogτS\" -> 0.000000000000   ,  \"σlogτN\" -> 0.000000000000   ,  \"σητ1\" -> 0.000000000000   ,  \"σητS \" -> 0.000000000000   ,  \"σητN\" -> 0.000000000000    |>   , \n\"IDS0366_210908_RAW_cal__ref_\" ->   <|    \"ζ\" -> 0.044599134979   ,  \"τ1\" -> 0.022455429279   ,  \"τS\" -> 0.023337915843   ,  \"τN\" -> 0.005128755710   ,  \"τC\" -> 0.001792889841   ,  \"κ0\" -> 0.000000002649   ,  \"mm1\" -> 0.000071495516   ,  \"mm2\" -> 0.015101682830   ,  \"mm3\" -> 0.038811401254   ,  \"T\" -> 0.430000000000   ,  \"B\" -> 12.000000000000   ,  \"θ\" -> 60.000000000000   ,  \"Reoff\" -> 0.000000000000   ,  \"Imoff\" -> 0.000000000000   ,  \"στ1\" -> 0.000015607545   ,  \"στS\" -> 0.000001063228   ,  \"στN\" -> 0.000002022209   ,  \"τ11 \" -> 0.000000000000   ,  \"τ12\" -> 0.000000000000   ,  \"τ22\" -> 0.000000000000   ,  \"τN1\" -> 0.000000000000   ,  \"τN2\" -> 0.000000000000   ,  \"σηlogτ1 \" -> 0.040328561350   ,  \"σηlogτS\" -> 0.000330725156   ,  \"σηlogτN\" -> 0.044548205014   ,  \"σlogτ1\" -> 0.000695045482   ,  \"σlogτS\" -> 0.000045557962   ,  \"σlogτN\" -> 0.000394288447   ,  \"σητ1\" -> 0.000905595157   ,  \"σητS \" -> 0.000007718436   ,  \"σητN\" -> 0.000228476861    |>   , \n\"IDS0366_210908_RAW_cal__sam_\" ->   <|    \"ζ\" -> 0.029143715364   ,  \"τ1\" -> 0.026198855926   ,  \"τS\" -> 0.029745373312   ,  \"τN\" -> 0.006649011545   ,  \"τC\" -> 0.003090491846   ,  \"κ0\" -> 0.000000002869   ,  \"mm1\" -> 0.000079676072   ,  \"mm2\" -> 0.018163106475   ,  \"mm3\" -> 0.048501617675   ,  \"T\" -> 0.430000000000   ,  \"B\" -> 12.000000000000   ,  \"θ\" -> 60.000000000000   ,  \"Reoff\" -> -2237951.807228915390   ,  \"Imoff\" -> 0.000000000000   ,  \"στ1\" -> 0.000000000000   ,  \"στS\" -> 0.000000000000   ,  \"στN\" -> 0.000000000000   ,  \"τ11 \" -> 0.000000000000   ,  \"τ12\" -> 0.000000000000   ,  \"τ22\" -> 0.000000000000   ,  \"τN1\" -> 0.000000000000   ,  \"τN2\" -> 0.000000000000   ,  \"σηlogτ1 \" -> 0.000000000000   ,  \"σηlogτS\" -> 0.000000000000   ,  \"σηlogτN\" -> 0.000000000000   ,  \"σlogτ1\" -> 0.000000000000   ,  \"σlogτS\" -> 0.000000000000   ,  \"σlogτN\" -> 0.000000000000   ,  \"σητ1\" -> 0.000000000000   ,  \"σητS \" -> 0.000000000000   ,  \"σητN\" -> 0.000000000000    |>   , \n\"IDS0367_210908_RAW_cal__ref_\" ->   <|    \"ζ\" -> 0.034740009221   ,  \"τ1\" -> 0.017028751834   ,  \"τS\" -> 0.022162435410   ,  \"τN\" -> 0.002809238258   ,  \"τC\" -> 0.001913219314   ,  \"κ0\" -> 0.000000003308   ,  \"mm1\" -> 0.000059427665   ,  \"mm2\" -> 0.013533798262   ,  \"mm3\" -> 0.031187935063   ,  \"T\" -> 0.530000000000   ,  \"B\" -> 12.000000000000   ,  \"θ\" -> 60.000000000000   ,  \"Reoff\" -> 0.000000000000   ,  \"Imoff\" -> 0.000000000000   ,  \"στ1\" -> 0.000027033003   ,  \"στS\" -> 0.000001554115   ,  \"στN\" -> 0.000002352999   ,  \"τ11 \" -> 0.000000000000   ,  \"τ12\" -> 0.000000000000   ,  \"τ22\" -> 0.000000000000   ,  \"τN1\" -> 0.000000000000   ,  \"τN2\" -> 0.000000000000   ,  \"σηlogτ1 \" -> 0.045416924257   ,  \"σηlogτS\" -> 0.000278228215   ,  \"σηlogτN\" -> 0.045395504019   ,  \"σlogτ1\" -> 0.001587491763   ,  \"σlogτS\" -> 0.000070123814   ,  \"σlogτN\" -> 0.000837593181   ,  \"σητ1\" -> 0.000773393532   ,  \"σητS \" -> 0.000006166215   ,  \"σητN\" -> 0.000127526787    |>   , \n\"IDS0367_210908_RAW_cal__sam_\" ->   <|    \"ζ\" -> 0.024637271207   ,  \"τ1\" -> 0.025634847148   ,  \"τS\" -> 0.027302474030   ,  \"τN\" -> 0.003538185279   ,  \"τC\" -> 0.003933377133   ,  \"κ0\" -> 0.000000003566   ,  \"mm1\" -> 0.000083131278   ,  \"mm2\" -> 0.019726981228   ,  \"mm3\" -> 0.041358600771   ,  \"T\" -> 0.530000000000   ,  \"B\" -> 12.000000000000   ,  \"θ\" -> 60.000000000000   ,  \"Reoff\" -> -1629518.072289161380   ,  \"Imoff\" -> 0.000000000000   ,  \"στ1\" -> 0.000000000000   ,  \"στS\" -> 0.000000000000   ,  \"στN\" -> 0.000000000000   ,  \"τ11 \" -> 0.000000000000   ,  \"τ12\" -> 0.000000000000   ,  \"τ22\" -> 0.000000000000   ,  \"τN1\" -> 0.000000000000   ,  \"τN2\" -> 0.000000000000   ,  \"σηlogτ1 \" -> 0.000000000000   ,  \"σηlogτS\" -> 0.000000000000   ,  \"σηlogτN\" -> 0.000000000000   ,  \"σlogτ1\" -> 0.000000000000   ,  \"σlogτS\" -> 0.000000000000   ,  \"σlogτN\" -> 0.000000000000   ,  \"σητ1\" -> 0.000000000000   ,  \"σητS \" -> 0.000000000000   ,  \"σητN\" -> 0.000000000000    |>   , \n\"IDS0368_210908_RAW_cal__ref_\" ->   <|    \"ζ\" -> 0.027231595728   ,  \"τ1\" -> 0.015050030834   ,  \"τS\" -> 0.020840826339   ,  \"τN\" -> 0.001677171050   ,  \"τC\" -> 0.002801092038   ,  \"κ0\" -> 0.000000003924   ,  \"mm1\" -> 0.000065840915   ,  \"mm2\" -> 0.013031059806   ,  \"mm3\" -> 0.027885420541   ,  \"T\" -> 0.630000000000   ,  \"B\" -> 12.000000000000   ,  \"θ\" -> 60.000000000000   ,  \"Reoff\" -> 0.000000000000   ,  \"Imoff\" -> 0.000000000000   ,  \"στ1\" -> 0.000025618780   ,  \"στS\" -> 0.000001064388   ,  \"στN\" -> 0.000001464284   ,  \"τ11 \" -> 0.000000000000   ,  \"τ12\" -> 0.000000000000   ,  \"τ22\" -> 0.000000000000   ,  \"τN1\" -> 0.000000000000   ,  \"τN2\" -> 0.000000000000   ,  \"σηlogτ1 \" -> 0.047954951123   ,  \"σηlogτS\" -> 0.000209073519   ,  \"σηlogτN\" -> 0.045696441574   ,  \"σlogτ1\" -> 0.001702241050   ,  \"σlogτS\" -> 0.000051072269   ,  \"σlogτN\" -> 0.000873068059   ,  \"σητ1\" -> 0.000721723493   ,  \"σητS \" -> 0.000004357265   ,  \"σητN\" -> 0.000076640749    |>   , \n\"IDS0368_210908_RAW_cal__sam_\" ->   <|    \"ζ\" -> 0.021420270760   ,  \"τ1\" -> 0.018208454683   ,  \"τS\" -> 0.024985612374   ,  \"τN\" -> 0.002144760910   ,  \"τC\" -> 0.004931614434   ,  \"κ0\" -> 0.000000004254   ,  \"mm1\" -> 0.000086915042   ,  \"mm2\" -> 0.015826314138   ,  \"mm3\" -> 0.034938353162   ,  \"T\" -> 0.630000000000   ,  \"B\" -> 12.000000000000   ,  \"θ\" -> 60.000000000000   ,  \"Reoff\" -> -1204819.277108438310   ,  \"Imoff\" -> 0.000000000000   ,  \"στ1\" -> 0.000000000000   ,  \"στS\" -> 0.000000000000   ,  \"στN\" -> 0.000000000000   ,  \"τ11 \" -> 0.000000000000   ,  \"τ12\" -> 0.000000000000   ,  \"τ22\" -> 0.000000000000   ,  \"τN1\" -> 0.000000000000   ,  \"τN2\" -> 0.000000000000   ,  \"σηlogτ1 \" -> 0.000000000000   ,  \"σηlogτS\" -> 0.000000000000   ,  \"σηlogτN\" -> 0.000000000000   ,  \"σlogτ1\" -> 0.000000000000   ,  \"σlogτS\" -> 0.000000000000   ,  \"σlogτN\" -> 0.000000000000   ,  \"σητ1\" -> 0.000000000000   ,  \"σητS \" -> 0.000000000000   ,  \"σητN\" -> 0.000000000000    |>   , \n\"IDS0369_210908_RAW_cal__ref_\" ->   <|    \"ζ\" -> 0.020332946442   ,  \"τ1\" -> 0.011808248331   ,  \"τS\" -> 0.019124131146   ,  \"τN\" -> 0.000708402175   ,  \"τC\" -> 0.003056309257   ,  \"κ0\" -> 0.000000005441   ,  \"mm1\" -> 0.000052779905   ,  \"mm2\" -> 0.011105332134   ,  \"mm3\" -> 0.023942232708   ,  \"T\" -> 0.830000000000   ,  \"B\" -> 12.000000000000   ,  \"θ\" -> 60.000000000000   ,  \"Reoff\" -> 0.000000000000   ,  \"Imoff\" -> 0.000000000000   ,  \"στ1\" -> 0.000047094116   ,  \"στS\" -> 0.000001159219   ,  \"στN\" -> 0.000001405585   ,  \"τ11 \" -> 0.000000000000   ,  \"τ12\" -> 0.000000000000   ,  \"τ22\" -> 0.000000000000   ,  \"τN1\" -> 0.000000000000   ,  \"τN2\" -> 0.000000000000   ,  \"σηlogτ1 \" -> 0.053002916420   ,  \"σηlogτS\" -> 0.000126082533   ,  \"σηlogτN\" -> 0.046399219380   ,  \"σlogτ1\" -> 0.003988238919   ,  \"σlogτS\" -> 0.000060615502   ,  \"σlogτN\" -> 0.001984162345   ,  \"σητ1\" -> 0.000625871599   ,  \"σητS \" -> 0.000002411219   ,  \"σητN\" -> 0.000032869308    |>   , \n\"IDS0369_210908_RAW_cal__sam_\" ->   <|    \"ζ\" -> 0.014606512986   ,  \"τ1\" -> 0.019756664879   ,  \"τS\" -> 0.022303249954   ,  \"τN\" -> 0.001023812506   ,  \"τC\" -> 0.005490022400   ,  \"κ0\" -> 0.000000005866   ,  \"mm1\" -> 0.000063747249   ,  \"mm2\" -> 0.017921258799   ,  \"mm3\" -> 0.030929470731   ,  \"T\" -> 0.830000000000   ,  \"B\" -> 12.000000000000   ,  \"θ\" -> 60.000000000000   ,  \"Reoff\" -> -481927.710843376814   ,  \"Imoff\" -> 0.000000000000   ,  \"στ1\" -> 0.000000000000   ,  \"στS\" -> 0.000000000000   ,  \"στN\" -> 0.000000000000   ,  \"τ11 \" -> 0.000000000000   ,  \"τ12\" -> 0.000000000000   ,  \"τ22\" -> 0.000000000000   ,  \"τN1\" -> 0.000000000000   ,  \"τN2\" -> 0.000000000000   ,  \"σηlogτ1 \" -> 0.000000000000   ,  \"σηlogτS\" -> 0.000000000000   ,  \"σηlogτN\" -> 0.000000000000   ,  \"σlogτ1\" -> 0.000000000000   ,  \"σlogτS\" -> 0.000000000000   ,  \"σlogτN\" -> 0.000000000000   ,  \"σητ1\" -> 0.000000000000   ,  \"σητS \" -> 0.000000000000   ,  \"σητN\" -> 0.000000000000    |>   , \n\"IDS0370_210908_RAW_cal__ref_\" ->   <|    \"ζ\" -> 0.016443978585   ,  \"τ1\" -> 0.012644854996   ,  \"τS\" -> 0.017634511441   ,  \"τN\" -> 0.000316227766   ,  \"τC\" -> 0.002708386911   ,  \"κ0\" -> 0.000000007589   ,  \"mm1\" -> 0.000038134808   ,  \"mm2\" -> 0.012179834504   ,  \"mm3\" -> 0.021381193373   ,  \"T\" -> 1.130000000000   ,  \"B\" -> 12.000000000000   ,  \"θ\" -> 60.000000000000   ,  \"Reoff\" -> 0.000000000000   ,  \"Imoff\" -> 0.000000000000   ,  \"στ1\" -> 0.000121213865   ,  \"στS\" -> 0.000001160231   ,  \"στN\" -> 0.000001536991   ,  \"τ11 \" -> 0.000000000000   ,  \"τ12\" -> 0.000000000000   ,  \"τ22\" -> 0.000000000000   ,  \"τN1\" -> 0.000000000000   ,  \"τN2\" -> 0.000000000000   ,  \"σηlogτ1 \" -> 0.048314482275   ,  \"σηlogτS\" -> 0.000048505756   ,  \"σηlogτN\" -> 0.045503358655   ,  \"σlogτ1\" -> 0.009586022574   ,  \"σlogτS\" -> 0.000065793194   ,  \"σlogτN\" -> 0.004860390947   ,  \"σητ1\" -> 
